vi "tsapp_disconnect.vi"(8 "error in (no error)":errorcluster, 11 "Path":path) -> (0 "error output":errorcluster, 2 "retuen":i32, 3 "Path output":path)   [LabVIEW 2014]
doc: "Function Introduction：\nDisconnect the device connection\nCall location：\nNo need to use hardware devices, call this function to disconnect the device connection\ninput parameter \nnothing\nReturn value ：\n==0: Device disconnected successfully\nOther values, query error code"
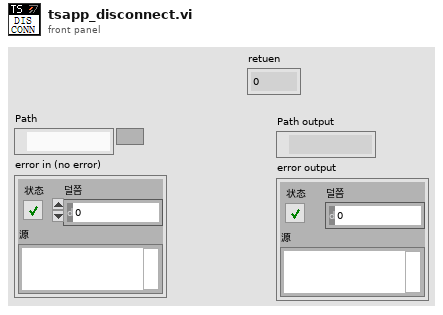
[diagram p1: front panel]
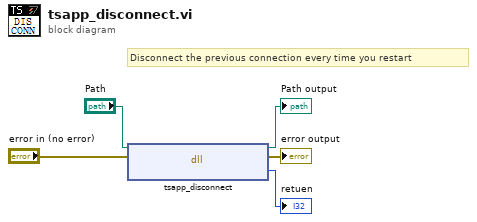
[diagram p0: block diagram]
diagram:
  # "Disconnect the previous connection every time you restart"
  n1 = dll-call lib="PTH2Zabs CUsers\nAdministratorDesktopLB2018TS_CAN通讯 文件夹PathTSMaster.dll" fn="tsapp_disconnect"(path in="Path", error in="error in (no error)") -> (path out=→"Path output":path, error out=→"error output":errorcluster, "tsapp_disconnect"=→"retuen":i32)  [unwired: 1 in]
